vi "createLoopArray.vi"(0 "Bgstop":dbl, 1 "Bgstop2":dbl, 2 "nbpoint1":dbl, 3 "nbpoint2":dbl, 4 "Bgstart":dbl) -> (5 "Outarray":dbl[](array[numeric]))   [LabVIEW 2011]
uses:
  <vilib>/imath/engines/lvmath2/RunTimeEngine/ErrorHandling/NIMS_Finalize Error.vi
  <vilib>/imath/engines/lvmath2/RunTimeEngine/Managers/WorkSpace/UID Generator.vi
  <vilib>/imath/engines/lvmath2/RunTimeEngine/Managers/SymbolTable/Clear UID.vi
  <vilib>/imath/engines/lvmath2/RunTimeEngine/NodeEndStatement/NIMS_NodeEndStatement_Output.vi
  <instcachedir>/0/NIMS_NodeEndStatement_Output_53EC0D466D134D7ABD903AC30B43404B.lvgen/NIMS_NodeEndStatement_Output_53EC0D466D134D7ABD903AC30B43404B_001.vi
  <vilib>/imath/engines/lvmath2/RunTimeEngine/RunTimeType/NIMS_RunTimeType_From StrictType (excl LVString).vi
  <instcachedir>/0/NIMS_RunTimeType_From StrictType (excl LVString)_46AE8B54A11948F0BCCEB8091EE7AA4C.lvgen/NIMS_RunTimeType_From StrictType (excl LVString)_46AE8B54A11948F0BCCEB8091EE7AA4C_000.vi
  <vilib>/imath/engines/lvmath2/RunTimeEngine/LocalVariableDefStatement/MC_LocalVariableDefStatement_Display.vi
  <vilib>/imath/engines/lvmath2/RunTimeEngine/Managers/SymbolTable/NIMS_WorkSpace.lvlib
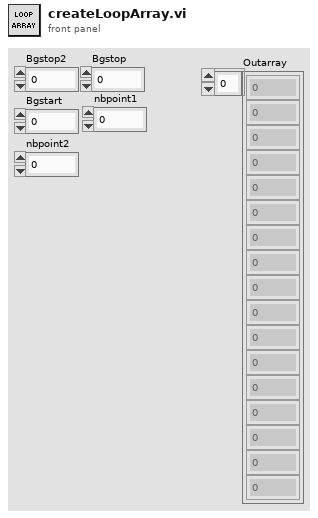
[diagram p1: front panel]
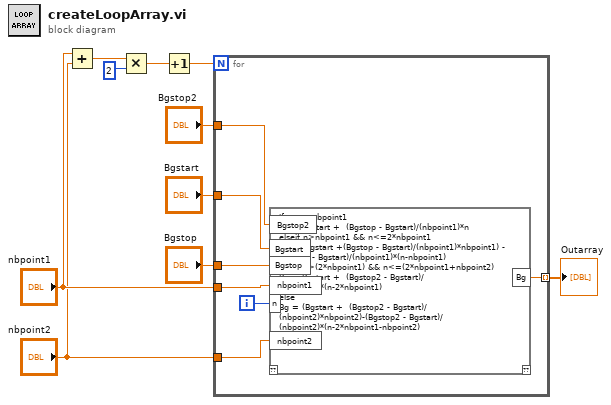
[diagram p0: block diagram]
diagram:
  n1 = Add(x="nbpoint1", y="nbpoint2") -> (x+y=w6:dbl)
  n2 = Multiply(x=w6, y=2) -> (x*y=w2:dbl)
  n3 = Increment(x=w2) -> (x+1=w1:dbl)
  n4 = for {
    N: w1 -> [_]
    tunnel: "Bgstop2" -> [w17]
    tunnel: "Bgstart" -> [w16]
    tunnel: "Bgstop" -> [w15]
    tunnel: "nbpoint1" -> [w14]
    tunnel: "nbpoint2" -> [w13]
    tunnel: [w12] -> w5 mode=indexing
    i -> [w11]
    n5 = mathscript code="if n <= nbpoint1 \nBg = Bgstart +  (Bgstop - Bgstart)/(nbpoint1)*n\nelseif n>nbpoint1 && n<=2*nbpoint1\nBg = (Bgstart +(Bgstop - Bgstart)/(nbpoint1)*nbpoint1) -  (Bgstop - Bgstart)/(nbpoint1)*(n-nbpoint1)\nelseif n>(2*nbpoint1) && n<=(2*nbpoint1+nbpoint2)\nBg = Bgstart +  (Bgstop2 - Bgstart)/(nbpoint2)*(n-2*nbpoint1)\nelse\nBg = (Bgstart +  (Bgstop2 - Bgstart)/(nbpoint2)*nbpoint2)-(Bgstop2 - Bgstart)/(nbpoint2)*(n-2*nbpoint1-nbpoint2)\nend"("Bgstart"=w16, "Bgstop"=w15, "nbpoint1"=w14, "n"=w11, "nbpoint2"=w13, "Bgstop2"=w17) -> ("Bg"=w12:dbl)  [unwired: 2 out]
  }
  "Outarray" <- w5
